vi "dq to abc conversion floating.vi"(8 "cos":sgl, 9 "sin":sgl, 10 "q":sgl, 11 "d":sgl) -> (1 "c":sgl format="%.2f", 2 "b":sgl format="%.2f", 3 "a":sgl format="%.2f")   [LabVIEW 2015]
uses:
  <vilib>/rvi/Emulation/niFpgaGetClockAttributes.vi
  <vilib>/rvi/Emulation/niFpgaSctlEmulationGetInTimedLoop.vi
  <vilib>/rvi/Emulation/niFpgaEmulationReportErrorSimple.vi
  <vilib>/rvi/Emulation/niFpgaCriticalErrorInLSC.vi
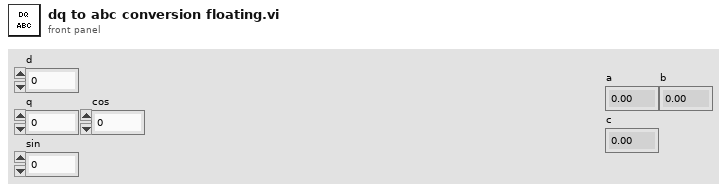
[diagram p1: front panel]
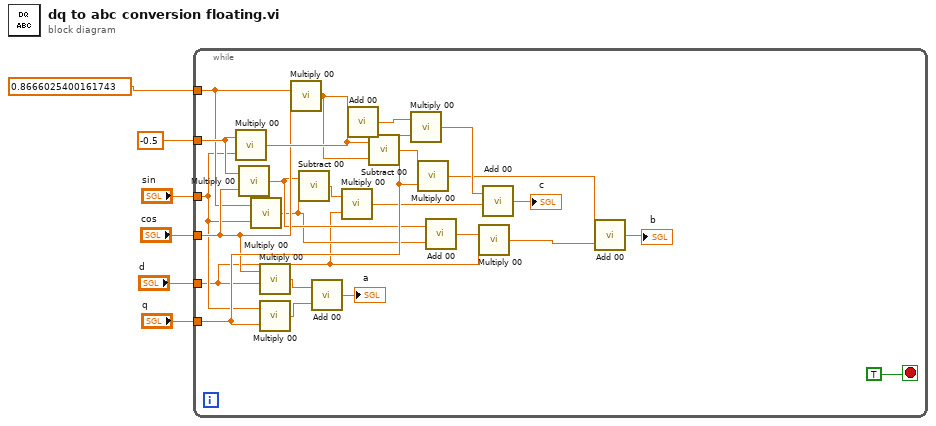
[diagram p0: block diagram]
diagram:
  n1 = while {
    tunnel: sgl 0.86660254 -> [w19]
    tunnel: "sin" -> [w18]
    tunnel: "cos" -> [w20]
    tunnel: sgl -0.5 -> [w21]
    tunnel: "d" -> [w10]
    tunnel: "q" -> [w22]
    stop <- TRUE stop-if-true
    n2 = call "Multiply 00.vi"("y"=w18, "x"=w21) -> ("x*y"=w25:sgl)
    n3 = call "Multiply 00.vi"("y"=w20, "x"=w21) -> ("x*y"=w13:sgl)
    n4 = call "Multiply 00.vi"("y"=w18, "x"=w19) -> ("x*y"=w12:sgl)
    n5 = call "Multiply 00.vi"("y"=w10, "x"=w20) -> ("x*y"=w29:sgl)
    n6 = call "Multiply 00.vi"("y"=w22, "x"=w18) -> ("x*y"=w28:sgl)
    n7 = call "Multiply 00.vi"("y"=w20, "x"=w19) -> ("x*y"=w24:sgl)
    n8 = call "Subtract 00.vi"("y"=w12, "x"=w13) -> ("x*y"=w17:sgl)
    n9 = call "Add 00.vi"("y"=w28, "x"=w29) -> ("x+y"=→"a":sgl)
    n10 = call "Multiply 00.vi"("y"=w10, "x"=w17) -> ("x*y"=w16:sgl)
    n11 = call "Add 00.vi"("y"=w25, "x"=w24) -> ("x+y"=w26:sgl)
    n12 = call "Subtract 00.vi"("y"=w24, "x"=w25) -> ("x*y"=w23:sgl)
    n13 = call "Multiply 00.vi"("y"=w22, "x"=w26) -> ("x*y"=w15:sgl)
    n14 = call "Multiply 00.vi"("y"=w22, "x"=w23) -> ("x*y"=w8:sgl)
    n15 = call "Add 00.vi"("y"=w12, "x"=w13) -> ("x+y"=w11:sgl)
    n16 = call "Multiply 00.vi"("y"=w10, "x"=w11) -> ("x*y"=w9:sgl)
    n17 = call "Add 00.vi"("y"=w16, "x"=w15) -> ("x+y"=→"c":sgl)
    n18 = call "Add 00.vi"("y"=w9, "x"=w8) -> ("x+y"=→"b":sgl)
  }
